vi "Update Files.vi"(10 "Step":refnum<vi>, 11 "WebView2 Updater in":refnum<class "WebView2 Updater.lvclass">) -> (0 "error out":errorcluster, 2 "Unzipped":bool)   [LabVIEW 2020, in "WebView2 Updater.lvclass"]
uses:
  WebView2 Updater.lvclass
  WebView2 Updater.lvclass/WebView2 Updater.ctl
  <vilib>/zip/NI_Unzip.lvlib
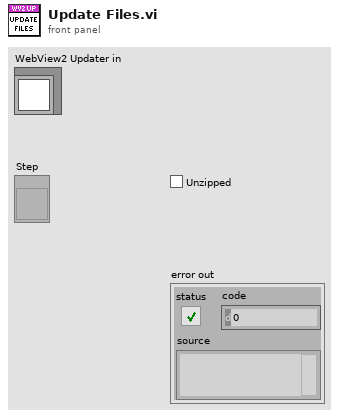
[diagram p1: front panel]
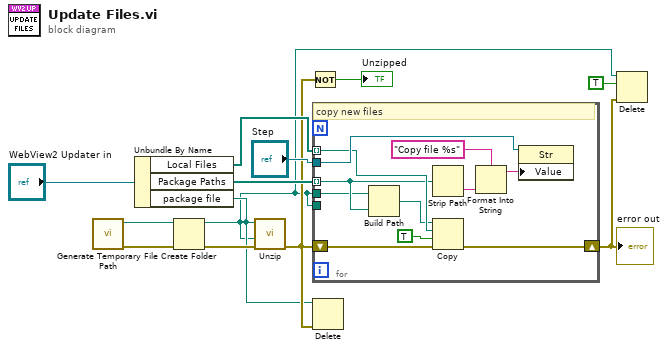
[diagram p0: block diagram]
diagram:
  n1 = call <vilib>:"Generate Temporary File Path.vi"() -> ("error out"=w6:errorcluster, "Unique Temporary File Path"=w8:path)  [unwired: 10 in]
  n2 = Unbundle By Name("WebView2 Updater in") -> ("Local Files"=w12:path[], "Package Paths"=w11:path[], "package file"=w2:path)
  n3 = Create Folder(path (use dialog)=w8, error in=w6) -> (created path=w1:path, error out=w7:errorcluster)  [unwired: 1 in, 1 out]
  n4 = call <vilib>:"Unzip.vi"("error in (no error)"=w7, "Target directory (same as Zip file if empty)"=w1, "Zip file"=w2) -> ("error out"=w10:errorcluster)  [unwired: 6 in, 2 out]
  n5 = Not(x=w10) -> (.not. x?=→"Unzipped":bool)
  n6 = for {
    tunnel: w12 -> [w18] mode=indexing
    tunnel: w1 -> [_]
    tunnel: w11 -> [w16] mode=indexing
    shift-right: [w23] -> w3
    shift-left: w10 -> [w24]
    tunnel: "Step" -> [w20]
    tunnel: w1 -> [w15]
    # "copy new files"
    n7 = Build Path(base path=w15, name or relative path=w16) -> (appended path=w14:path)
    n8 = Strip Path(path=w16) -> (name=w21:string)  [unwired: 1 out]
    n9 = Copy(8:w24, 9:TRUE ("overwrite (F)"), 10:w18, 11:w14) -> (0:w23:errorcluster)  [unwired: 1 in, 2 out]
    n10 = Format Into String(format string="Copy file %s", w21) -> (resulting string=w19:string)  [unwired: 2 in, 1 out]
    n11 = property class="Str"(reference=w20, "Value"=w19) -> ()  [unwired: 1 in, 2 out]
  }
  "error out" <- w3
  n12 = Delete(path (use dialog)=w2, error in=w10) -> ()  [unwired: 3 in, 3 out]
  n13 = Delete(path (use dialog)=w1, entire hierarchy (F)=TRUE, error in=w3) -> ()  [unwired: 2 in, 3 out]
